vi "__initialize_dependencies.vi"() -> ()   [LabVIEW 2020]
uses:
  <vilib>/AppBuilder/AB_API_Simple/Build (path).vi
  <vilib>/AppBuilder/AB_API_Simple/NI_App_Builder_API.lvlib
panel:
  out "String":string
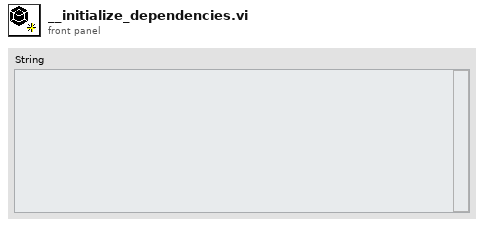
[diagram p1: front panel]
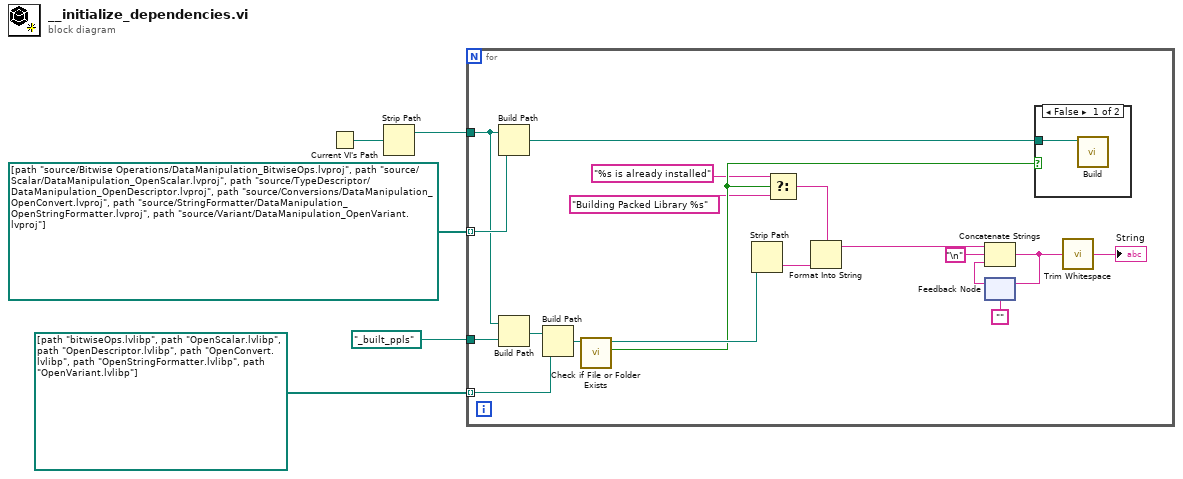
[diagram p0: block diagram]
diagram:
  n1 = Current VI's Path() -> (path=w5:path)
  n2 = Strip Path(path=w5) -> (stripped path=w4:path)  [unwired: 1 out]
  n3 = for {
    tunnel: w4 -> [w23]
    tunnel: path[] [path "source/Bitwise Operations/DataManipulation_BitwiseOps.lvproj", path "source/Scalar/DataManipulation_OpenScalar.lvproj", path "source/TypeDescriptor/DataManipulation_OpenDescriptor.lvproj", path "source/Conversions/DataManipulation_OpenConvert.lvproj", path "source/StringFormatter/DataManipulation_OpenStringFormatter.lvproj", path "source/Variant/DataManipulation_OpenVariant.lvproj"] -> [w24] mode=indexing
    tunnel: path "_built_ppls" -> [w22]
    tunnel: path[] [path "bitwiseOps.lvlibp", path "OpenScalar.lvlibp", path "OpenDescriptor.lvlibp", path "OpenConvert.lvlibp", path "OpenStringFormatter.lvlibp", path "OpenVariant.lvlibp"] -> [w20] mode=indexing
    n4 = Build Path(base path=w23, name or relative path=w24) -> (appended path=w11:path)
    n5 = Build Path(base path=w23, name or relative path=w22) -> (appended path=w21:path)
    n6 = Build Path(base path=w21, name or relative path=w20) -> (appended path=w19:path)
    n7 = call <vilib>:"Check if File or Folder Exists.vi"("path"=w19) -> ("file or folder exists?"=w9:bool, "dup path"=w18:path)  [unwired: 8 in, 1 out]
    n8 = Strip Path(path=w18) -> (name=w10:string)  [unwired: 1 out]
    n9 = Select(t="%s is already installed" ("format string"), s=w9, f="Building Packed Library %s" ("format string")) -> (s? t:f=w6:string)
    n10 = Format Into String(format string=w6, w10) -> (resulting string=w16:string)  [unwired: 2 in, 1 out]
    n11 = feedback #1("") -> (w12:string)
    n12 = Concatenate Strings(w16, "\n", w12) -> (w15:string)
    n13 = feedback-in #1(w15) -> ()
    n14 = case shown="False" w9 {
      tunnel: w11 -> [w25 _]
      frame False {
        n15 = call-poly <vilib>:"Build.vi"("Path to project"=w25) -> ()  [unwired: 9 in, 2 out]
      }
      frame True {
      }
    }
    n16 = call <vilib>:"Trim Whitespace.vi"("string"=w15) -> ("trimmed string"=→"String":string)  [unwired: 1 in]
  }
